vi "Configure Multi Eval Meas Limit Equalizer Spectrum Flatness.vi"(0 "VISA resource name":refnum<visa-resource-name>, 1 "Range 1 (6.0)":dbl=6.0 format="%^.3e", 2 "Max1 Min2 (7.0)":dbl=7.0 format="%^.3e", 5 "Instance (1)":T1=1, 7 "Modulation (Pi/2-BPSK)":i32(ring) items=["Pi/2-BPSK", "QPSK", "16-QAM", "64-QAM", "256-QAM"], 9 "Enable (On)":bool=TRUE, 11 "error in (no error)":errorcluster, 12 "Range 2 (9.0)":dbl=9.0 format="%^.3e", 13 "Max2 Min1 (8.0)":dbl=8.0 format="%^.3e") -> (4 "VISA resource name out":refnum<visa-resource-name>, 15 "error out":errorcluster)   [LabVIEW 2020, in "Rohde&Schwarz CMXP NR FR2 Measurement.lvlib"]
doc: "Defines limits for the equalizer spectrum flatness.\n\nAttributes:\nRSCMXPNRFR2M_ATTR_MULTI_EVAL_MEASUREMENT_LIMIT_PHBPSK_EQUALIZER_SPECTRUM_FLATNESS\nRSCMXPNRFR2M_ATTR_MULTI_EVAL_MEASUREMENT_LIMIT_QPSK_EQUALIZER_SPECTRUM_FLATNESS\nRSCMXPNRFR2M_ATTR_MULTI_EVAL_MEASUREMENT_LIMIT_QAM16_EQUALIZER_SPECTRUM_FLATNESS\nRSCMXPNRFR2M_ATTR_MULTI_EVAL_MEASUREMENT_LIMIT_QAM64_EQUALIZER_SPECTRUM_FLATNESS\nRSCMXPNRFR2M_ATTR_MULTI_EVAL_MEASUREMENT_LIMIT_QAM256_EQUALIZER_SPECTRUM_FLATNESS\n\nRemote-control commands:\nCONFigure:NRMMw:MEAS<i>:MEValuation:LIMit:PHBPsk:ESFLatness\nCONFigure:NRMMw:MEAS<i>:MEValuation:LIMit:QPSK:ESFLatness\nCONFigure:NRMMw:MEAS<i>:MEValuation:LIMit:QAM<order>:ESFLatness"
uses:
  <instrlib>/Rohde&Schwarz CMXP NR FR2 Measurement/Rohde&Schwarz CMXP NR FR2 Measurement.lvlib
  <instrlib>/Rohde&Schwarz CMXP NR FR2 Measurement/Private/_Instance.ctl
  <instrlib>/Rohde&Schwarz CMXP NR FR2 Measurement/Private/rsidr_core.llb/rsidr_core.lvlib
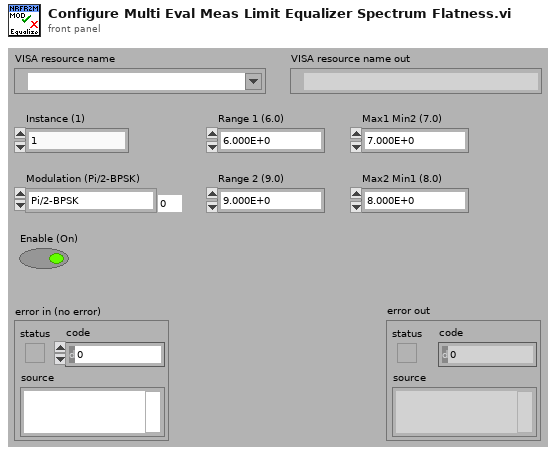
[diagram p1: front panel]
types:
  T1 = typedef "Rohde&Schwarz CMXP NR FR2 Measurement.lvlib/_Instance.ctl" = i32
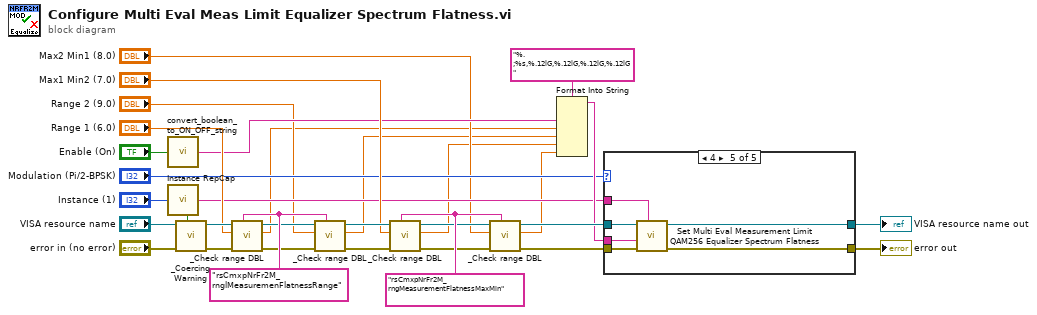
[diagram p0: block diagram]
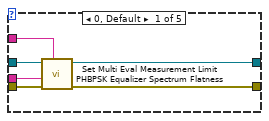
[diagram p2: hidden frame]
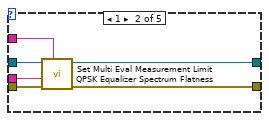
[diagram p3: hidden frame]
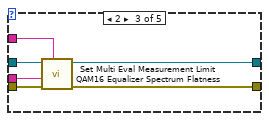
[diagram p4: hidden frame]
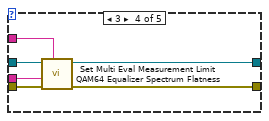
[diagram p5: hidden frame]
diagram:
  w22 = "rsCmxpNrFr2M_rngMeasurementFlatnessMaxMin"
  w26 = "rsCmxpNrFr2M_rnglMeasuremenFlatnessRange"
  n1 = call <instrlib>:"convert_boolean_to_ON_OFF_string.vi"("boolean value in"="Enable (On)") -> ("string value out"=w15:string)  [unwired: 4 in]
  n2 = call <instrlib>:"Instance RepCap.vi"("Instance In"="Instance (1)") -> ("In Range?"=w29:bool, "RepCap Identifier Out"=w11:string)  [unwired: 1 in]
  n3 = call <instrlib>:"_Coercing Warning.vi"("In Range?"=w29, "error in (no error)"="error in (no error)", "VISA resource name"="VISA resource name") -> ("error out"=w28:errorcluster, "VISA resource name out"=w27:refnum<visa-resource-name>)  [unwired: 7 in]
  n4 = call <instrlib>:"_Check range DBL.vi"("Range Table Identifier"=w26, "error in (no error)"=w28, "DBL Value In"="Range 1 (6.0)", "VISA resource name"=w27) -> ("error out"=w23:errorcluster, "DBL Value Out"=w5:dbl, "VISA resource name out"=w24:refnum<visa-resource-name>)  [unwired: 5 in]
  n5 = call <instrlib>:"_Check range DBL.vi"("Range Table Identifier"=w26, "error in (no error)"=w23, "DBL Value In"="Range 2 (9.0)", "VISA resource name"=w24) -> ("error out"=w20:errorcluster, "DBL Value Out"=w4:dbl, "VISA resource name out"=w21:refnum<visa-resource-name>)  [unwired: 5 in]
  n6 = call <instrlib>:"_Check range DBL.vi"("Range Table Identifier"=w22, "error in (no error)"=w20, "DBL Value In"="Max1 Min2 (7.0)", "VISA resource name"=w21) -> ("error out"=w17:errorcluster, "DBL Value Out"=w3:dbl, "VISA resource name out"=w18:refnum<visa-resource-name>)  [unwired: 5 in]
  n7 = call <instrlib>:"_Check range DBL.vi"("Range Table Identifier"=w22, "error in (no error)"=w17, "DBL Value In"="Max2 Min1 (8.0)", "VISA resource name"=w18) -> ("error out"=w14:errorcluster, "DBL Value Out"=w2:dbl, "VISA resource name out"=w13:refnum<visa-resource-name>)  [unwired: 5 in]
  n8 = Format Into String(format string="%.;%s,%.12lG,%.12lG,%.12lG,%.12lG", w15, w5, w4, w3, w2) -> (resulting string=w12:string)  [unwired: 2 in, 1 out]
  n9 = case shown="4" "Modulation (Pi/2-BPSK)" {
    tunnel: w14 -> [w38 w44 w50 w56 w62]
    tunnel: w13 -> [w37 w43 w49 w55 w61]
    tunnel: w12 -> [w33 w39 w45 w51 w57]
    tunnel: w11 -> [w36 w42 w48 w54 w60]
    tunnel: [w35 w41 w47 w53 w59] -> w8
    tunnel: [w34 w40 w46 w52 w58] -> w9
    frame 0, Default {
      n10 = call "Set Multi Eval Measurement Limit PHBPSK Equalizer Spectrum Flatness"("Repeated Capabilities"=w36, "error in (no error)"=w38, "Multi Eval Measurement Limit PHBPSK Equalizer Spectrum Flatness ()"=w33, "instrument handle"=w37) -> ("error out"=w35:errorcluster, "instrument handle out"=w34:refnum<visa-resource-name>)  [unwired: 6 in]
    }
    frame 1 {
      n11 = call "Set Multi Eval Measurement Limit QPSK Equalizer Spectrum Flatness"("Repeated Capabilities"=w42, "error in (no error)"=w44, "Multi Eval Measurement Limit QPSK Equalizer Spectrum Flatness ()"=w39, "instrument handle"=w43) -> ("error out"=w41:errorcluster, "instrument handle out"=w40:refnum<visa-resource-name>)  [unwired: 6 in]
    }
    frame 2 {
      n12 = call "Set Multi Eval Measurement Limit QAM16 Equalizer Spectrum Flatness"("Repeated Capabilities"=w48, "error in (no error)"=w50, "Multi Eval Measurement Limit QAM16 Equalizer Spectrum Flatness ()"=w45, "instrument handle"=w49) -> ("error out"=w47:errorcluster, "instrument handle out"=w46:refnum<visa-resource-name>)  [unwired: 6 in]
    }
    frame 3 {
      n13 = call "Set Multi Eval Measurement Limit QAM64 Equalizer Spectrum Flatness"("Repeated Capabilities"=w54, "error in (no error)"=w56, "Multi Eval Measurement Limit QAM64 Equalizer Spectrum Flatness ()"=w51, "instrument handle"=w55) -> ("error out"=w53:errorcluster, "instrument handle out"=w52:refnum<visa-resource-name>)  [unwired: 6 in]
    }
    frame 4 {
      n14 = call "Set Multi Eval Measurement Limit QAM256 Equalizer Spectrum Flatness"("Repeated Capabilities"=w60, "error in (no error)"=w62, "Multi Eval Measurement Limit QAM256 Equalizer Spectrum Flatness ()"=w57, "instrument handle"=w61) -> ("error out"=w59:errorcluster, "instrument handle out"=w58:refnum<visa-resource-name>)  [unwired: 6 in]
    }
  }
  "error out" <- w8
  "VISA resource name out" <- w9
